vi "Set_VXM_Home_win7.vi"(1 "error in (no error)":errorcluster) -> (0 "error out":errorcluster)   [LabVIEW 2017]
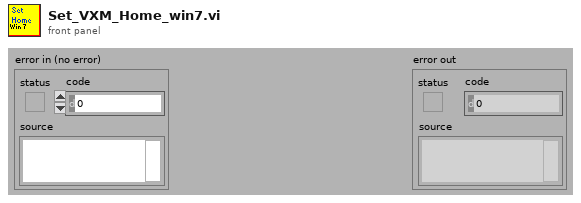
[diagram p1: front panel]
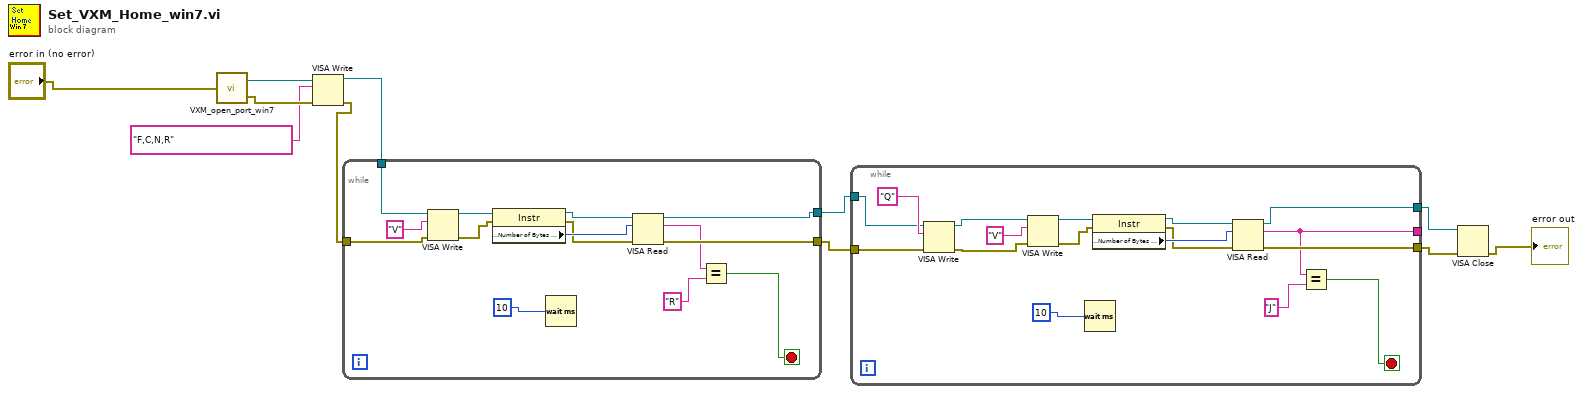
[diagram p0: block diagram]
diagram:
  n1 = call "VXM_open_port_win7.vi"("error in (no error)"="error in (no error)") -> ("VISA resource name out"=w11:refnum<visa-resource-name>, "error out"=w10:errorcluster)
  n2 = VISA Write(VISA resource name=w11, write buffer="F,C,N,R", error in (no error)=w10) -> (VISA resource name out=w5:refnum<visa-resource-name>, error out=w6:errorcluster)  [unwired: 1 out]
  n3 = while {
    tunnel: w6 -> [w22]
    tunnel: w5 -> [w21]
    tunnel: [w17] -> w3
    tunnel: [w12] -> w4
    stop <- w14 stop-if-true
    n4 = VISA Write(VISA resource name=w21, write buffer="V", error in (no error)=w22) -> (VISA resource name out=w24:refnum<visa-resource-name>, error out=w23:errorcluster)  [unwired: 1 out]
    n5 = property class="Instr"(reference=w24, error in=w23) -> (reference out=w19:refnum<visa-resource-name>, error out=w18:errorcluster, "Serial Settings:Number of Bytes at Serial Port"=w20:u32)
    n6 = Wait (ms)(milliseconds to wait=10) -> ()  [unwired: 1 out]
    n7 = VISA Read(VISA resource name=w19, byte count=w20, error in (no error)=w18) -> (VISA resource name out=w12:refnum<visa-resource-name>, read buffer=w15:string, error out=w17:errorcluster)  [unwired: 1 out]
    n8 = Equal?(x=w15, y="R") -> (x = y?=w14:bool)
  }
  n9 = while {
    tunnel: [w33] -> _
    tunnel: [w36] -> w2
    tunnel: [w35] -> w1
    tunnel: w4 -> [w28]
    tunnel: w3 -> [w29]
    stop <- w32 stop-if-true
    n10 = VISA Write(VISA resource name=w28, write buffer="Q", error in (no error)=w29) -> (VISA resource name out=w27:refnum<visa-resource-name>, error out=w26:errorcluster)  [unwired: 1 out]
    n11 = VISA Write(VISA resource name=w27, write buffer="V", error in (no error)=w26) -> (VISA resource name out=w41:refnum<visa-resource-name>, error out=w40:errorcluster)  [unwired: 1 out]
    n12 = Wait (ms)(milliseconds to wait=10) -> ()  [unwired: 1 out]
    n13 = property class="Instr"(reference=w41, error in=w40) -> (reference out=w38:refnum<visa-resource-name>, error out=w37:errorcluster, "Serial Settings:Number of Bytes at Serial Port"=w39:u32)
    n14 = VISA Read(VISA resource name=w38, byte count=w39, error in (no error)=w37) -> (VISA resource name out=w36:refnum<visa-resource-name>, read buffer=w33:string, error out=w35:errorcluster)  [unwired: 1 out]
    n15 = Equal?(x=w33, y="J") -> (x = y?=w32:bool)
  }
  n16 = VISA Close(VISA resource name=w2, error in (no error)=w1) -> (error out=→"error out":errorcluster)
